vi "Open Image.vi"(8 "error in (no error)":errorcluster, 11 "EmbedImage in":refnum<class "EmbedImage.lvclass">) -> (0 "error out":errorcluster, 3 "EmbedImage out":refnum<class "EmbedImage.lvclass">)   [LabVIEW 2023, in "EmbedImage.lvlib" / "EmbedImage.lvclass"]
uses:
  Library/EmbedImage.lvclass
  Library/EmbedImage.lvclass/EmbedImage.ctl
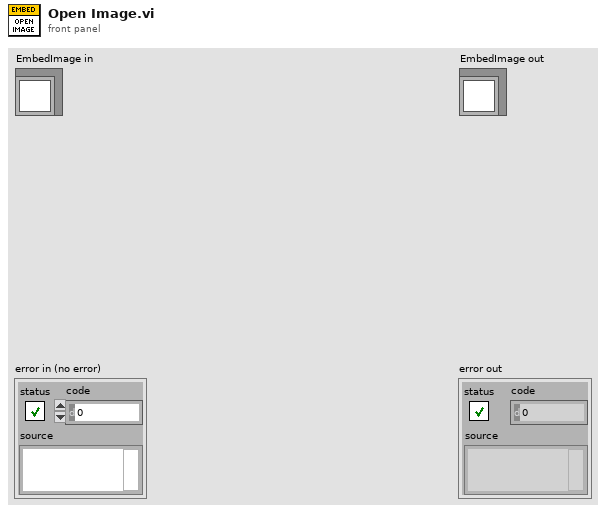
[diagram p1: front panel]
types:
  T1 = typedef "EmbedImage.lvlib/EmbedImage.lvclass/Image Types.ctl" = enum16{"PNG", "JPG", "JPEG", "BMP"}
  T2 = typedef "imagedata.ctl" = cluster{"image type":i32, "image depth":i32, "image":u8[], "mask":u8[], "colors":u32[], "Rectangle":cluster{"left":i16, "top":i16, "right":i16, "bottom":i16}}
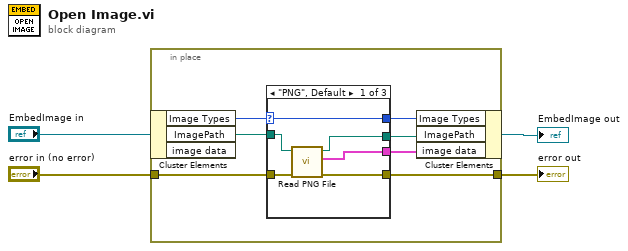
[diagram p0: block diagram]
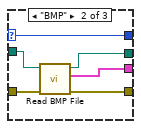
[diagram p2: hidden frame]
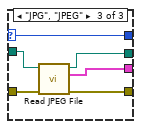
[diagram p3: hidden frame]
diagram:
  n1 = in-place {
    in-place-border: "error in (no error)" -> [w6]
    in-place-border: [w5] -> w1
    n2 = in-place-cluster #1("EmbedImage in") -> ("Image Types"=w11:T1, "ImagePath"=w10:path)  [unwired: 1 out]
    n3 = case shown="\"PNG\", Default" w11 {
      selector: w11 -> [w15 w23 w27]
      tunnel: w10 -> [w17 w22 w29]
      tunnel: [w16 w21 w28] -> w9
      tunnel: [w15 w23 w27] -> w8
      tunnel: [w14 w20 w26] -> w7
      tunnel: w6 -> [w13 w19 w25]
      tunnel: [w12 w18 w24] -> w5
      frame "PNG", Default {
        n4 = call <vilib>:"Read PNG File.vi"("error in (no error)"=w13, "path to PNG file"=w17) -> ("error out"=w12:errorcluster, "image data"=w14:T2, "path"=w16:path)  [unwired: 7 in]
      }
      frame "BMP" {
        n5 = call <vilib>:"Read BMP File.vi"("error in (no error)"=w19, "path to BMP file"=w22) -> ("error out"=w18:errorcluster, "image data"=w20:T2, "path"=w21:path)  [unwired: 7 in]
      }
      frame "JPG", "JPEG" {
        n6 = call <vilib>:"Read JPEG File.vi"("error in (no error)"=w25, "path to JPEG file"=w29) -> ("error out"=w24:errorcluster, "image data"=w26:T2, "path"=w28:path)  [unwired: 7 in]
      }
    }
    n7 = in-place-cluster #1("Image Types"=w8, "ImagePath"=w9, "image data"=w7) -> (→"EmbedImage out":refnum<class "EmbedImage.lvclass">)
  }
  "error out" <- w1
